vi "Fetch Multi Eval Meas List Segment ACLR Results.vi"(6 "Segment (1)":T3=1, 8 "error in (no error)":errorcluster, 9 "Result Type (Current)":i32(ring) items=["Current", "Average"], 10 "Instance (1)":T4=1, 11 "VISA resource name":refnum<visa-resource-name>) -> (0 "error out":errorcluster, 1 "ACLR Results":T2 {"NR Positive" format="%^.3e"; "NR Negative" format="%^.3e"; "UTRA 2 Positive" format="%^.3e"; "UTRA 1 Positive" format="%^.3e"; "Carrier" format="%^.3e"; "UTRA 1 Negative" format="%^.3e"; "UTRA 2 Negative" format="%^.3e"}, 2 "Reliability Results":T1, 3 "VISA resource name out":refnum<visa-resource-name>, 4 "Expired Statistics":i32, 5 "Out Of Tolerance":i32)   [LabVIEW 2020, in "Rohde&Schwarz CMWXP NR FR1 Measurement.lvlib"]
doc: "Return ACLR single value results for segment <no> in list mode.\n\nAttributes:\nRSCMWXPNRFR1M_ATTR_FETCH_MULTI_EVAL_MEAS_LIST_SEGMENT_ACLR_CURRENT_RESULTS\nRSCMWXPNRFR1M_ATTR_FETCH_MULTI_EVAL_MEAS_LIST_SEGMENT_ACLR_AVERAGE_RESULTS\n\nRemote-control commands:\nFETCh:NRSub:MEAS<i>:MEValuation:LIST:SEGMent<no>:ACLR:CURRent?\nFETCh:NRSub:MEAS<i>:MEValuation:LIST:SEGMent<no>:ACLR:AVERage?"
uses:
  <instrlib>/Rohde&Schwarz CMWXP NR FR1 Measurement/Rohde&Schwarz CMWXP NR FR1 Measurement.lvlib
  <instrlib>/Rohde&Schwarz CMWXP NR FR1 Measurement/Private/_Instance.ctl
  <instrlib>/Rohde&Schwarz CMWXP NR FR1 Measurement/Private/_Segment.ctl
  <instrlib>/Rohde&Schwarz CMWXP NR FR1 Measurement/Private/_SegReliability.ctl
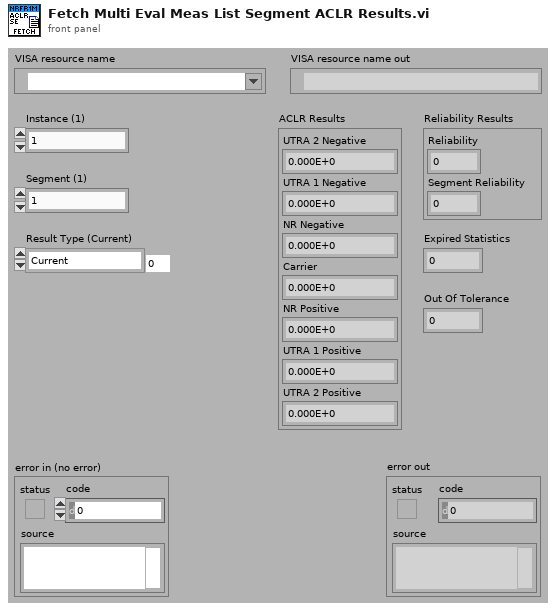
[diagram p1: front panel]
types:
  T1 = typedef "Rohde&Schwarz CMWXP NR FR1 Measurement.lvlib/_SegReliability.ctl" = cluster{"Reliability":i32, "Segment Reliability":i32}
  T2 = cluster{"UTRA 2 Negative":dbl, "UTRA 1 Negative":dbl, "NR Negative":dbl, "Carrier":dbl, "NR Positive":dbl, "UTRA 1 Positive":dbl, "UTRA 2 Positive":dbl}
  T3 = typedef "Rohde&Schwarz CMWXP NR FR1 Measurement.lvlib/_Segment.ctl" = i32
  T4 = typedef "Rohde&Schwarz CMWXP NR FR1 Measurement.lvlib/_Instance.ctl" = i32
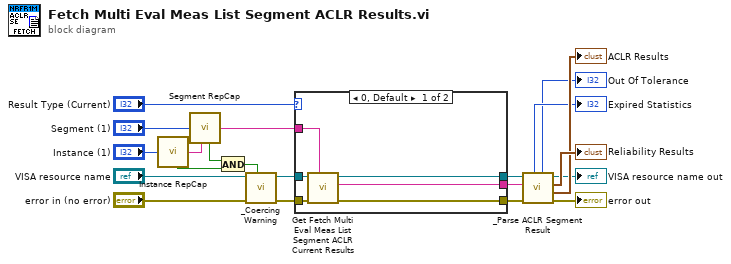
[diagram p0: block diagram]
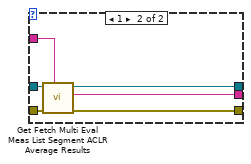
[diagram p2: hidden frame]
diagram:
  n1 = call <instrlib>:"Instance RepCap.vi"("Instance In"="Instance (1)") -> ("In Range?"=w17:bool, "RepCap Identifier Out"=w16:string)  [unwired: 1 in]
  n2 = call <instrlib>:"Segment RepCap.vi"("Segment In"="Segment (1)", "RepCap String In (\"\")"=w16) -> ("In Range?"=w15:bool, "RepCap Identifier Out"=w11:string)
  n3 = And(x=w15, y=w17) -> (x .and. y?=w19:bool)
  n4 = call <instrlib>:"_Coercing Warning.vi"("In Range?"=w19, "error in (no error)"="error in (no error)", "VISA resource name"="VISA resource name") -> ("error out"=w12:errorcluster, "VISA resource name out"=w13:refnum<visa-resource-name>)  [unwired: 7 in]
  n5 = case shown="0, Default" "Result Type (Current)" {
    tunnel: w13 -> [w27 w33]
    tunnel: w12 -> [w26 w32]
    tunnel: w11 -> [w25 w31]
    tunnel: [w24 w30] -> w9
    tunnel: [w23 w29] -> w8
    tunnel: [w22 w28] -> w7
    frame 0, Default {
      n6 = call "Get Fetch Multi Eval Meas List Segment ACLR Current Results"("Repeated Capabilities"=w25, "error in (no error)"=w26, "instrument handle"=w27) -> ("error out"=w22:errorcluster, "Fetch Multi Eval Meas List Segment ACLR Current Results"=w23:string, "instrument handle out"=w24:refnum<visa-resource-name>)  [unwired: 6 in]
    }
    frame 1 {
      n7 = call "Get Fetch Multi Eval Meas List Segment ACLR Average Results"("Repeated Capabilities"=w31, "error in (no error)"=w32, "instrument handle"=w33) -> ("error out"=w28:errorcluster, "Fetch Multi Eval Meas List Segment ACLR Average Results"=w29:string, "instrument handle out"=w30:refnum<visa-resource-name>)  [unwired: 6 in]
    }
  }
  n8 = call <instrlib>:"_Parse ACLR Segment Result.vi"("error in (no error)"=w7, "Input String"=w8, "VISA resource name"=w9) -> ("error out"=→"error out":errorcluster, "ACLR Results"=→"ACLR Results":T2, "Reliability Results"=→"Reliability Results":T1, "VISA resource name out"=→"VISA resource name out":refnum<visa-resource-name>, "Out Of Tolerance"=→"Out Of Tolerance":i32, "Statistic Expired"=→"Expired Statistics":i32)  [unwired: 3 in]
